vi "FTW-Ether-CreatePublisher.vi"(5 "Requested Publisher Address":string, 11 "error in":errorcluster) -> (4 "Publisher Endpoint":refnum<class "FTW-Endpoint.lvclass">, 6 "Actual Publisher Address":string, 15 "error out":errorcluster)   [LabVIEW 2013, in "FTW-Ether.lvclass"]
uses:
  FTW-Ether.lvclass
  Endpoint/FTW-Endpoint.lvclass
  FTW-Ether-EndpointType.ctl
panel:
  # "Inputs"
  # "Outputs"
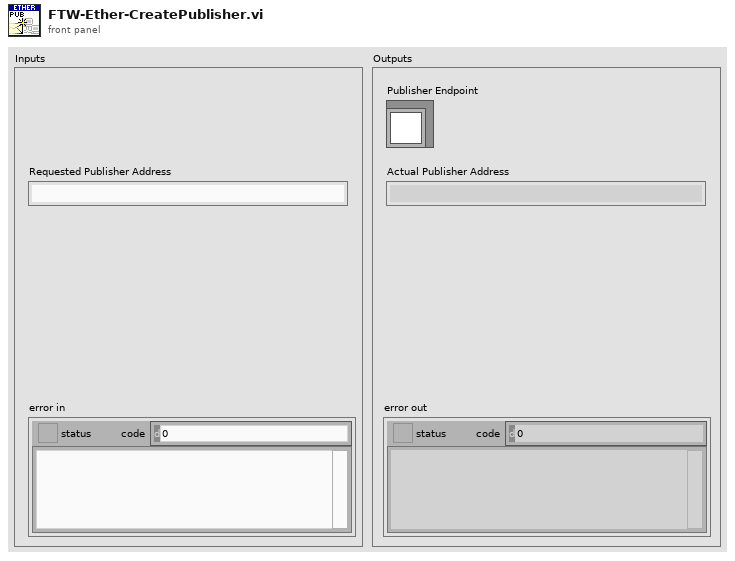
[diagram p1: front panel]
types:
  T1 = typedef "FTW-Ether.lvclass/FTW-Ether-EndpointType.ctl" = enum16{"Server", "Client", "Publisher", "Subscriber"}
  T2 = typedef "FTW-Ether.lvclass/FTW-Ether-MessageTransportScheme.ctl" = enum16{"LabVIEW Queues (lvq://)", "LabVIEW Notifiers (lvn://)", "LabVIEW Network Streams (lvns://)"}
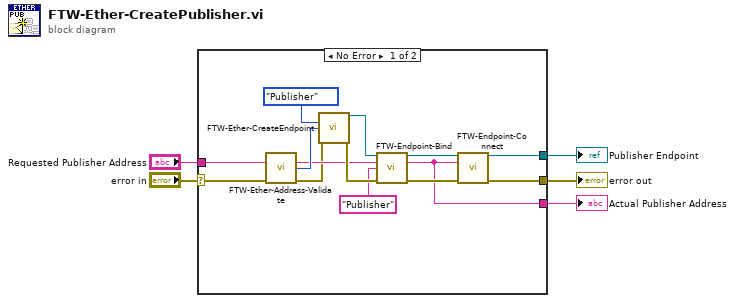
[diagram p0: block diagram]
diagram:
  n1 = case shown="No Error" "error in" {
    selector: "error in" -> [w11 w20]
    tunnel: [w18 _] -> w2
    tunnel: [w17 w20] -> w3
    tunnel: [w12 _] -> w4
    tunnel: "Requested Publisher Address" -> [w7 _]
    frame No Error {
      n2 = call "FTW-Ether-Address-Validate.vi"("Address"=w7, "error in"=w11) -> ("Sanitized Address"=w9:string, "Message Transport Scheme"=w10:T2, "error out"=w8:errorcluster)  [unwired: 11 in]
      n3 = call "FTW-Ether-CreateEndpoint.vi"("Endpoint Type"=FTW-Ether-EndpointType."Publisher", "Message Transport Scheme"=w10, "error in"=w8) -> ("FTW Endpoint"=w16:refnum<class "FTW-Endpoint.lvclass">, "error out"=w14:errorcluster)  [unwired: 11 in]
      n4 = call-dynamic "FTW-Endpoint-Bind.vi"("FTW Endpoint"=w16, "Endpoint Address"=w9, "Requested Identity"="Publisher", "error in"=w14) -> ("FTW Endpoint out"=w15:refnum<class "FTW-Endpoint.lvclass">, "Actual Endpoint Address"=w12:string, "error out"=w13:errorcluster)  [unwired: 8 in, 1 out]
      n5 = call-dynamic "FTW-Endpoint-Connect.vi"("FTW Endpoint"=w15, "Endpoint Address"=w12, "error in"=w13) -> ("FTW Endpoint out"=w18:refnum<class "FTW-Endpoint.lvclass">, "error out"=w17:errorcluster)  [unwired: 11 in]
    }
    frame Error {
    }
  }
  "error out" <- w3
  "Publisher Endpoint" <- w2
  "Actual Publisher Address" <- w4
